vi "Stop Core.vi"(10 "final error code":i32, 11 "UI Status in":refnum<class "UI Status.lvclass">) -> (3 "UI Status out":refnum<class "UI Status.lvclass">)   [LabVIEW 2020, in "UI Status.lvlib" / "UI Status.lvclass"]
doc: "(<B>Filename</B>: Actor Framework.lvlib:Actor.lvclass:Stop Core.vi)\n\nDefines what the actor does before it stops. Use the <B>final error code</B> input to determine whether the actor shut down in response to an error.\n\nBy default, this method passes the Stop message along to all auto-stop nested actors. A descendant class may override this method to define additional behavior, such as shutting down any processes the actor initiated in its override of the Actor Core method."
uses:
  UI Status.lvclass
  UI Status.lvclass/UI Status.ctl
  <vilib>/ActorFramework/Actor/Actor.lvclass
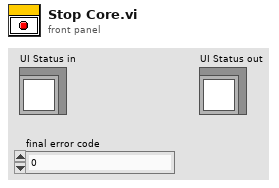
[diagram p1: front panel]
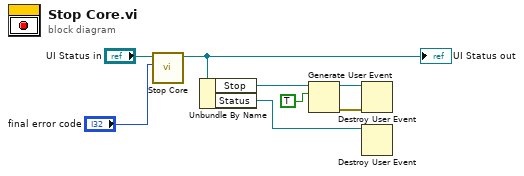
[diagram p0: block diagram]
diagram:
  n1 = call-parent "Stop Core.vi"("final error code"="final error code", "Actor in"="UI Status in") -> ("Actor out"=w6:refnum<class "UI Status.lvclass">)  [unwired: 9 in]
  "UI Status out" <- w6
  n2 = Unbundle By Name(w6) -> ("Stop"=w5:refnum<user-event>, "Status"=w1:refnum<user-event>)
  n3 = Generate User Event(user event=w5, event data cluster=TRUE ("event data")) -> (user event out=w2:refnum<user-event>, error out=w3:errorcluster)  [unwired: 2 in]
  n4 = Destroy User Event(user event=w2, error in=w3) -> ()  [unwired: 1 out]
  n5 = Destroy User Event(user event=w1) -> ()  [unwired: 1 in, 1 out]
